vi "Workers 4.0 Debug Server EXE Launcher.vi"(8 "error in (no error)":errorcluster) -> (0 "error out":errorcluster)   [LabVIEW 2017, in "Application Manager.lvclass"]
doc: "Run the Workers 4.0 Debug Server applicaiton EXE"
uses:
  Application Manager/Application Manager.lvclass
  <vilib>/Utility/sysdir.llb/System Directory Type.ctl
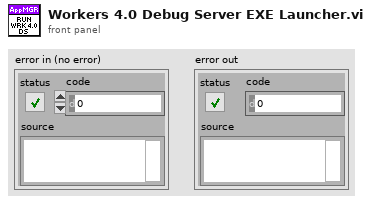
[diagram p1: front panel]
types:
  T1 = typedef "System Directory Type.ctl" = i32
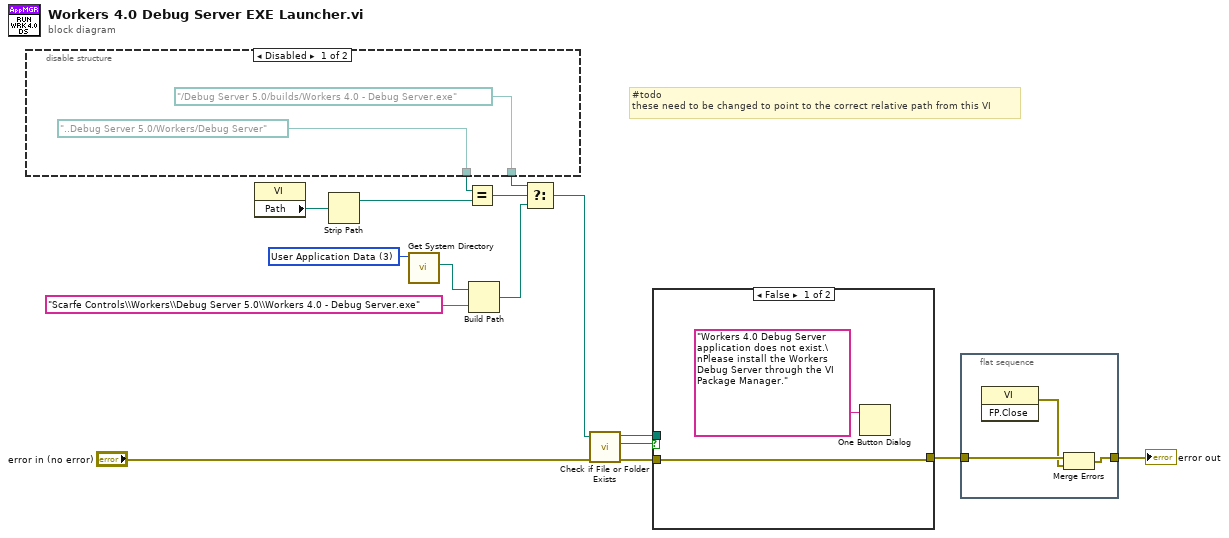
[diagram p0: block diagram]
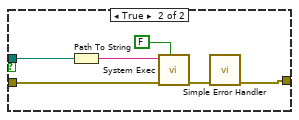
[diagram p3: hidden frame]
diagram:
  w12 = T1 3 items=["User Home"=0, "User Desktop"=1, "User Documents"=2, "User Application Data"=3, "User Preferences"=4, "User Temporary"=5, "Public Documents"=6, "Public Application Data"=7, "Public Preferences"=8, "Public Cache"=13, "System Core Libraries"=9, "System Installed Libraries"=10, "Application Files"=11, "Boot Volume Root"=12] ("system directory type")
  # "#todo\nthese need to be changed to point to the correct relative path from this VI"
  n1 = disable-structure shown="Disabled" {
    disable-tunnel: [path "..Debug Server 5.0/Workers/Debug Server" _] -> w10
    disable-tunnel: [path "../Debug Server 5.0/builds/Workers 4.0 - Debug Server.exe" _] -> w8
    frame Disabled {
    }
    frame Enabled {
    }
  }
  n2 = property class="VI"() -> ("Path"=w2:path)  [unwired: 2 in, 2 out]
  n3 = Strip Path(path=w2) -> (stripped path=w1:path)  [unwired: 1 out]
  n4 = call <vilib>:"Get System Directory.vi"("system directory type"=w12) -> ("system directory"=w11:path)  [unwired: 10 in]
  n5 = Equal?(x=w10, y=w1) -> (x = y?=w9:bool)
  n6 = Build Path(base path=w11, name or relative path="Scarfe Controls\\Workers\\Debug Server 5.0\\Workers 4.0 - Debug Server.exe") -> (appended path=w7:path)
  n7 = Select(t=w8, s=w9, f=w7) -> (s? t:f=w5:path)
  n8 = call <vilib>:"Check if File or Folder Exists.vi"("error in (no error)"="error in (no error)", "path"=w5) -> ("error out"=w6:errorcluster, "file or folder exists?"=w3:bool, "dup path"=w4:path)  [unwired: 7 in]
  n9 = case shown="False" w3 {
    tunnel: [w20 w26] -> w14
    tunnel: w6 -> [w20 w22]
    tunnel: w4 -> [_ w21]
    frame False {
      n10 = One Button Dialog(message="Workers 4.0 Debug Server application does not exist.\nPlease install the Workers Debug Server through the VI Package Manager.") -> ()  [unwired: 1 in, 1 out]
    }
    frame True {
      n11 = Path To String(path=w21) -> (string=w23:string)
      n12 = call <vilib>:"System Exec.vi"("wait until completion? (T)"=FALSE, "error in (no error)"=w22, "command line"=w23) -> ("error out"=w25:errorcluster)  [unwired: 5 in, 3 out]
      n13 = call <vilib>:"Simple Error Handler.vi"("error in (no error)"=w25) -> ("error out"=w26:errorcluster)  [unwired: 4 in, 4 out]
    }
  }
  n14 = flat-sequence {
    tunnel: [w28] -> w15
    tunnel: w14 -> [w29]
    frame #0 {
      n15 = invoke class="VI" method="FP.Close"() -> (error out=w27:errorcluster)  [unwired: 3 in, 2 out]
      n16 = Merge Errors(w29, w27) -> (w28:errorcluster)
    }
  }
  "error out" <- w15
